vi "DSF.Shared.Configuration.Transfer.Set Channel Descriptors.vi"(8 "error in (no error)":errorcluster, 10 "Channel Descriptors":T1[](array[typedef]) {"VS Channel Ref" format="%016x"; "Channel Parameters"."offset" format="%d bytes"}, 11 "Transfer Configuration in":refnum<class "DSF.Shared.Configuration.Transfer.lvclass">) -> (0 "error out":errorcluster, 3 "Transfer Configuration out":refnum<class "DSF.Shared.Configuration.Transfer.lvclass">)   [LabVIEW 2016, in "DSF.Shared.lvlib" / "DSF.Shared.Configuration.Transfer.lvclass"]
uses:
  DSF.Shared.Configuration.Transfer.lvclass
  Typedefs/DSF.Shared.Typedefs.Configuration.Transfer.Channel Descriptor.ctl
  Typedefs/DSF.Shared.Typedefs.Configuration.Transfer.Channel Parameters.ctl
  Typedefs/DSF.Shared.Typedefs.Data Type.ctl
  <vilib>/NI Veristand/Custom Device API/Custom Device Item Ref.ctl
  DSF.Shared.Configuration.Transfer.lvclass/DSF.Shared.Configuration.Transfer.ctl
  VIs/DSF.Shared.Data Type.Sizeof.vi
  DSF.Shared.Configuration.Transfer.Channel Descriptors Equal.vi
  DSF.Shared.Configuration.Transfer.Check.Channel Parameters.Contiguous.vi
  DSF.Shared.Configuration.Transfer.Errors.vi
  DSF.Shared.Configuration.Transfer.Errors.Channels Not Contiguous.vi
  DSF.Shared.lvlib
  <vilib>/NI Veristand/Custom Device API/Custom Device API.lvlib
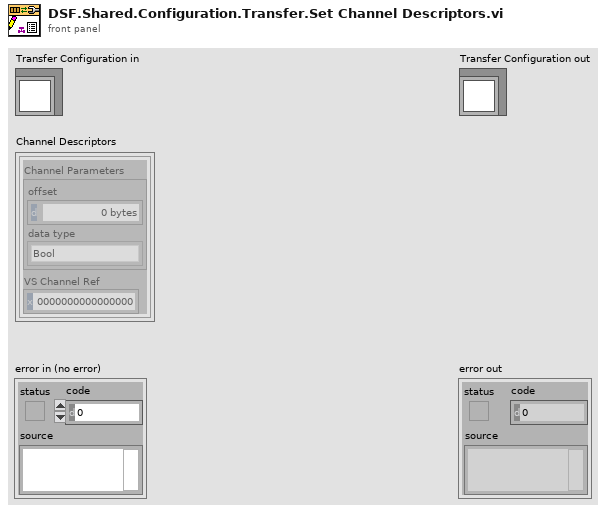
[diagram p1: front panel]
types:
  T1 = typedef "DSF.Shared.lvlib/DSF.Shared.Typedefs.Configuration.Transfer.Channel Descriptor.ctl" = cluster{"Channel Parameters":T2, "VS Channel Ref":T4}
  T2 = typedef "DSF.Shared.lvlib/DSF.Shared.Typedefs.Configuration.Transfer.Channel Parameters.ctl" = cluster{"offset":u64, "data type":T3}
  T3 = typedef "DSF.Shared.lvlib/DSF.Shared.Typedefs.Data Type.ctl" = enum8{"Bool", "SGL", "DBL", "I8", "I16", "I32", "I64", "U8", "U16", "U32", "U64"}
  T4 = typedef "Custom Device API.lvlib/Custom Device Item Ref.ctl" = u64
  T5 = typedef "DSF.Shared.lvlib/DSF.Shared.Typedefs.Configuration.Transfer.Channel Block Descriptor.ctl" = cluster{"First Channel Descriptor":T1, "count":u64, "vs channel index":u64}
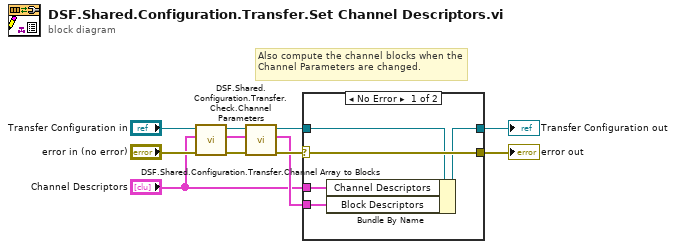
[diagram p0: block diagram]
diagram:
  # "Also compute the channel blocks when the Channel Parameters are changed."
  n1 = call "DSF.Shared.Configuration.Transfer.Check.Channel Parameters.vi"("error in (no error)"="error in (no error)", "Channel Parameters in"="Channel Descriptors", "Transfer Configuration in"="Transfer Configuration in") -> ("error out"=w3:errorcluster, "Channel Parameters out"=w1:T1[], "Transfer Configuration out"=w4:refnum<class "DSF.Shared.Configuration.Transfer.lvclass">)  [unwired: 6 in]
  n2 = call "DSF.Shared.Configuration.Transfer.Channel Array to Blocks.vi"("error in (no error)"=w3, "Channel Descriptors"=w1, "Transfer Configuration in"=w4) -> ("error out"=w9:errorcluster, "Channel Block Descriptors"=w7:T5[], "Transfer Configuration out"=w10:refnum<class "DSF.Shared.Configuration.Transfer.lvclass">)  [unwired: 6 in]
  n3 = case shown="No Error" w9 {
    selector: w9 -> [w16 w17]
    tunnel: "Channel Descriptors" -> [w15 _]
    tunnel: [w14 w18] -> w11
    tunnel: w10 -> [w13 w18]
    tunnel: w7 -> [w12 _]
    tunnel: [w16 w17] -> w8
    frame No Error {
      n4 = Bundle By Name(cluster=w13, "Channel Descriptors"=w15, "Block Descriptors"=w12) -> (w14:refnum<class "DSF.Shared.Configuration.Transfer.lvclass">)
    }
    frame Error {
    }
  }
  "error out" <- w8
  "Transfer Configuration out" <- w11
